vi "SerializeMessage.vi"(7 "MsgSerializer":refnum<class "MsgSerializer.lvclass">, 9 "error in (no error)":errorcluster, 10 "Value":variant, 11 "TestManagerMsg.Verbose in":refnum<class "TestManagerMsg.Verbose.lvclass">) -> (1 "error out":errorcluster, 3 "Serialized Message":string)   [LabVIEW 2013, in "Caraya.lvlib" / "TestManagerMsg.Verbose.lvclass"]
uses:
  TestManagerMsg.Verbose.lvclass
  MsgSerializer/MsgSerializer.lvclass
  TestManagerMsg.Verbose.lvclass/TestManagerMsg.Verbose.ctl
  Test Manager Message/TestManagerMsg.lvclass
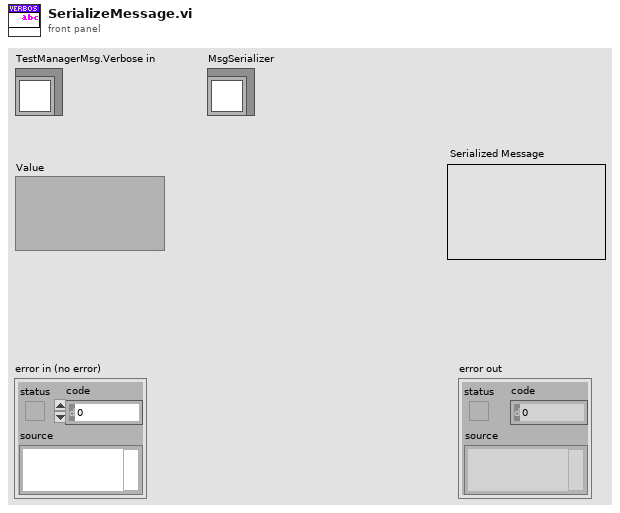
[diagram p1: front panel]
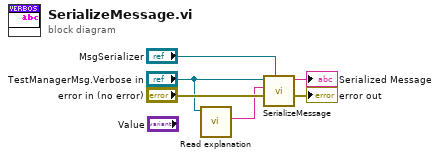
[diagram p0: block diagram]
diagram:
  n1 = call "Read explanation.vi"("TestManagerMsg.Verbose in"="TestManagerMsg.Verbose in") -> ("explanation"=w1:string)  [unwired: 9 in, 1 out]
  n2 = call-parent "SerializeMessage.vi"("MsgSerializer"="MsgSerializer", "error in (no error)"="error in (no error)", "Value"=w1, "TestManagerMsg in"="TestManagerMsg.Verbose in") -> ("error out"=→"error out":errorcluster, "Serialized Message"=→"Serialized Message":string)  [unwired: 6 in]
